vi "Update String Control Value By Name.vi"(6 "Disabled":T2(ring), 7 "Result":T1(ring), 8 "error in (no error)":errorcluster, 9 "Data":string, 10 "String Control Name":string(combo), 11 "Controls[]":refnum<vi>[](array[refnum])) -> (0 "error out":errorcluster, 2 "Specific Ref":refnum<vi>, 3 "Controls[] Out":refnum<vi>[](array[refnum]))   [LabVIEW 2021]
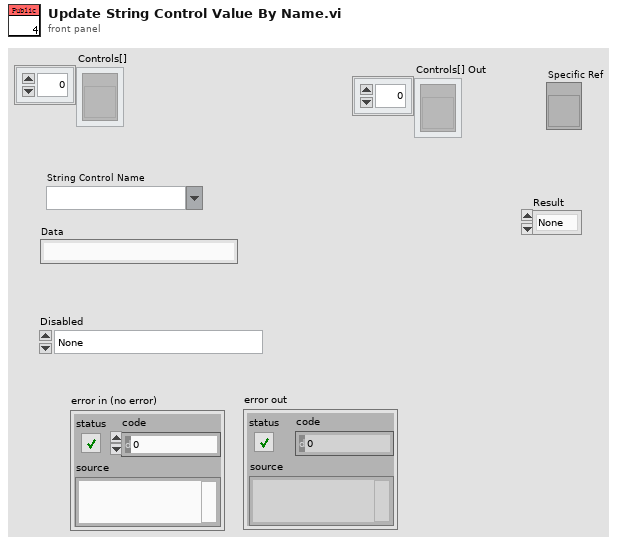
[diagram p1: front panel]
types:
  T1 = enum16{"None", "Initialize", "Testing", "OK", "NG"}
  T2 = enum8{"None", "Enabled", "Disabled", "Disabled and Grayed Out"}
  T3 = enum8{"Enabled", "Disabled", "Disabled and Grayed Out"}
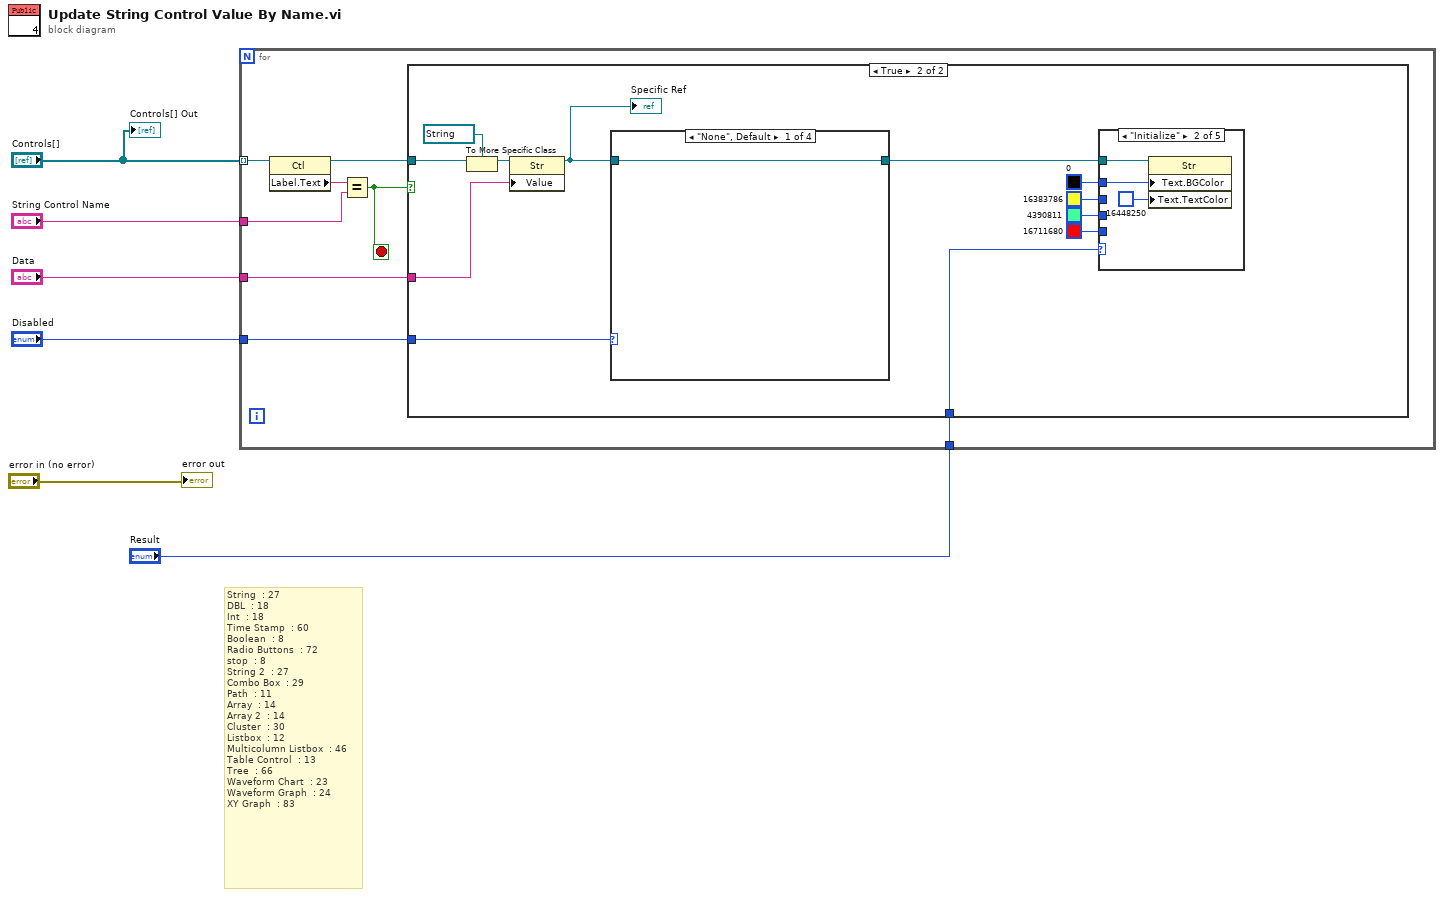
[diagram p0: block diagram]
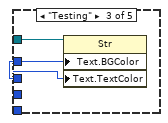
[diagram p4: hidden frame]
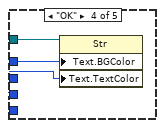
[diagram p5: hidden frame]
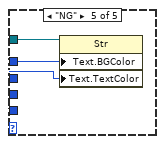
[diagram p6: hidden frame]
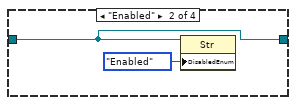
[diagram p7: hidden frame]
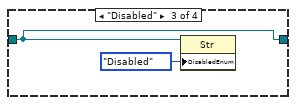
[diagram p8: hidden frame]
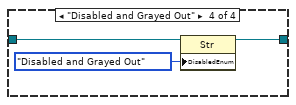
[diagram p9: hidden frame]
diagram:
  # "String  : 27\nDBL  : 18\nInt  : 18\nTime Stamp  : 60\nBoolean  : 8\nRadio Buttons  : 72\nstop  : 8\nString 2  : 27\nCombo Box  : 29\nPath  : 11\nArray  : 14\nArray 2  : 14\nCluster  : 30\nListbox  : 12\nMulticolumn Listbox  : 46\nTable Control  : 13\nTree  : 66\nWaveform Chart  : 23\nWaveform Graph  : 24\nXY Graph  : 83"
  n1 = for {
    tunnel: "Controls[]" -> [w14] mode=indexing
    tunnel: "String Control Name" -> [w12]
    tunnel: "Data" -> [w9]
    tunnel: "Disabled" -> [w8]
    tunnel: "Result" -> [w7]
    stop <- w11 stop-if-true
    n2 = property class="Ctl"(reference=w14) -> (reference out=w10:refnum<vi>, "Label.Text"=w13:string)  [unwired: 1 in, 1 out]
    n3 = Equal?(x=w13, y=w12) -> (x = y?=w11:bool)
    n4 = case shown="True" w11 {
      tunnel: w10 -> [_ w24]
      tunnel: w9 -> [_ w23]
      tunnel: w8 -> [_ w21]
      tunnel: w7 -> [_ w19]
      frame False {
      }
      frame True {
        n5 = To More Specific Class(target class=refnum<vi> refnum ("RoleName"), reference=w24) -> (specific class reference=w26:refnum<vi>)  [unwired: 1 in, 1 out]
        n6 = property class="Str"(reference=w26, "Value"=w23) -> (reference out=w22:refnum<vi>)  [unwired: 1 in, 1 out]
        "Specific Ref" <- w22
        n7 = case shown="\"None\", Default" w21 {
          tunnel: w22 -> [w39 w41 w43 w46]
          tunnel: [w39 w41 w43 w44] -> w20
          frame "None", Default {
          }
          frame "Enabled" {
            n8 = property class="Str"(reference=w41, "DisabledEnum"=T3."Enabled" ("Disabled")) -> ()  [unwired: 1 in, 2 out]
          }
          frame "Disabled" {
            n9 = property class="Str"(reference=w43, "DisabledEnum"=T3."Disabled" ("Disabled")) -> ()  [unwired: 1 in, 2 out]
          }
          frame "Disabled and Grayed Out" {
            n10 = property class="Str"(reference=w46, "DisabledEnum"=T3."Disabled and Grayed Out" ("Disabled")) -> (reference out=w44:refnum<vi>)  [unwired: 1 in, 1 out]
          }
        }
        n11 = case shown="\"Initialize\"" w19 {
          tunnel: w20 -> [_ w29 w32 w35 w38]
          tunnel: u32 0 ("Initialize") -> [_ w28 w30 w34 w37]
          tunnel: u32 16383786 ("Testing") -> [_ _ w31 _ _]
          tunnel: u32 4390811 ("OK") -> [_ _ _ w33 _]
          tunnel: u32 16711680 ("NG") -> [_ _ _ _ w36]
          frame "None", Default {
          }
          frame "Initialize" {
            n12 = property class="Str"(reference=w29, "Text.BGColor"=w28, "Text.TextColor"=u32 16448250 ("Testing")) -> ()  [unwired: 1 in, 2 out]
          }
          frame "Testing" {
            n13 = property class="Str"(reference=w32, "Text.BGColor"=w31, "Text.TextColor"=w30) -> ()  [unwired: 1 in, 2 out]
          }
          frame "OK" {
            n14 = property class="Str"(reference=w35, "Text.BGColor"=w33, "Text.TextColor"=w34) -> ()  [unwired: 1 in, 2 out]
          }
          frame "NG" {
            n15 = property class="Str"(reference=w38, "Text.BGColor"=w36, "Text.TextColor"=w37) -> ()  [unwired: 1 in, 2 out]
          }
        }
      }
    }
  }
  "error out" <- "error in (no error)"
  "Controls[] Out" <- "Controls[]"
